vi "Simplify Mathematical Equations.vi"() -> ()   [LabVIEW 2021]
panel:
  out "Simplified Equation":string
  in  "Input Equation":string
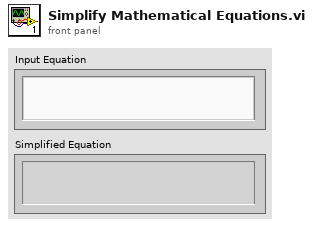
[diagram p1: front panel]
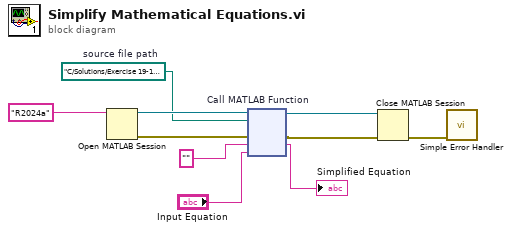
[diagram p0: block diagram]
diagram:
  w3 = path "C:/Solutions/Exercise 19-1 Simplifying Equations with MATLAB in NI LabVIEW/Simplify.m"  # source file path
  n1 = Open MATLAB Session(0:"R2024a" ("release name")) -> (8:w10:refnum<k37>, 11:w9:errorcluster)  [unwired: 1 in]
  n2 = node "Call MATLAB Function"(w10, w3, w9, "", "Input Equation") -> (w6:refnum<k37>, w7:errorcluster, →"Simplified Equation":string)  [unwired: 2 in, 2 out]
  n3 = Close MATLAB Session(0:w6, 3:w7) -> (11:w5:errorcluster)
  n4 = call <vilib>:"Simple Error Handler.vi"("error in (no error)"=w5) -> ()  [unwired: 4 in, 5 out]
